vi "Play Path.vi"(7 "Description":string, 8 "Command Info In":T5, 11 "Path stuff":T4 {"Limits"."Limits"."StoopidFast (fps)" min=0.0; "Limits"."Limits"."Jerk (fps^3)" min=0.0 step=1.0; "Limits"."Limits"."Accel (fps^2)" min=0.0; "Limits"."Limits"."Velocity (fps)" min=0.0}) -> (0 "Command Info Out":T5)   [LabVIEW 2019]
doc: "This VI notifies the subsystem to the new setpoint."
uses:
  <vilib>/Rock Robotics/WPI/Framework/Command Status Info.ctl
  <vilib>/Rock Robotics/WPI/Framework/Completion Status.ctl
  <vilib>/Rock Robotics/WPI/Framework/Completion Notifier.ctl
  Support Code/Single Cmd Info.ctl
  <vilib>/picture/picture.llb/imagedata.ctl
  Support Code/types/Limits.ctl
  Implementation/Drive Operations.ctl
  Implementation/Drive Setpoints.ctl
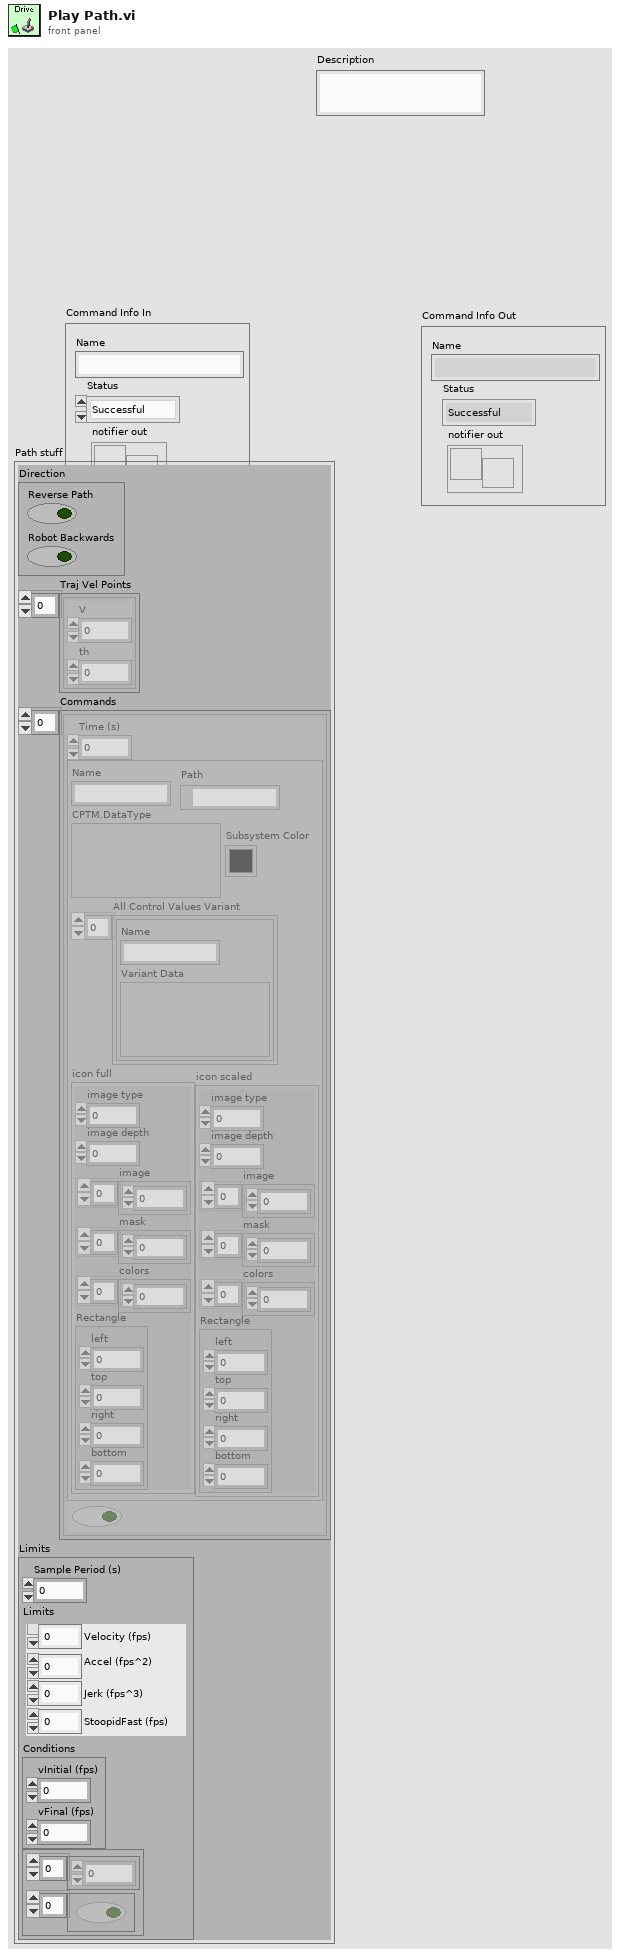
[diagram p1: front panel]
types:
  T1 = typedef "Single Cmd Info.ctl" = cluster{"Name":string, "CPTM.DataType":variant, "All Control Values Variant":cluster{"Name":string, "Variant Data":variant}[], "icon full":T2, "icon scaled":T2, "Path":path, "Subsystem Color":u32}
  T2 = typedef "imagedata.ctl" = cluster{"image type":i32, "image depth":i32, "image":u8[], "mask":u8[], "colors":u32[], "Rectangle":cluster{"left":i16, "top":i16, "right":i16, "bottom":i16}}
  T3 = typedef "Limits.ctl" = cluster{"Velocity (fps)":dbl, "Accel (fps^2)":dbl, "Jerk (fps^3)":dbl, "StoopidFast (fps)":dbl}
  T4 = cluster{"Direction":cluster{"Reverse Path":bool, "Robot Backwards":bool}, "Traj Vel Points":cluster{"V":dbl, "th":dbl}[], "Commands":cluster{"Time (s)":dbl, T1, bool}[], "Limits":cluster{"Sample Period (s)":dbl, "Limits":T3, "Conditions":cluster{"vInitial (fps)":dbl, "vFinal (fps)":dbl}, cluster{dbl[], bool[]}}}
  T5 = typedef "Command Status Info.ctl" = cluster{"Name":string, "Status":T6, "notifier out":T7}
  T6 = typedef "Completion Status.ctl" = enum16{"Successful", "Aborted", "Incomplete"}
  T7 = typedef "Completion Notifier.ctl" = refnum<notifier>
  T8 = typedef "Drive Operations.ctl" = enum16{"Reserve", "Read Current", "Immediate", "Play Path"}
  T9 = typedef "Drive Setpoints.ctl" = cluster{"Operation":T8, "Setpoints":cluster{"Left Setpoint":dbl, "Right Setpoint":dbl}, "Path stuff":cluster{"Direction":cluster{"Reverse Path":bool, "Robot Backwards":bool}, "Traj Vel Points":cluster{"V":dbl, "th":dbl}[], "Commands":cluster{"Time (s)":dbl, T1, bool}[], "Limits":cluster{"Sample Period (s)":dbl, "Limits":T3, "Conditions":cluster{"vInitial (fps)":dbl, "vFinal (fps)":dbl}, cluster{dbl[], bool[]}}}}
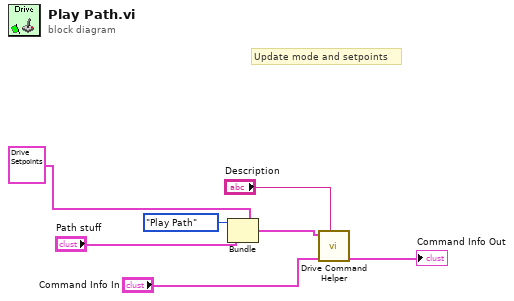
[diagram p0: block diagram]
diagram:
  # "Update mode and setpoints"
  n1 = Bundle(cluster=T9 {"Operation"=enum."Reserve", "Setpoints"={"Left Setpoint"=0.0, "Right Setpoint"=0.0}, "Path stuff"={"Direction"={"Reverse Path"=FALSE, "Robot Backwards"=FALSE}, "Traj Vel Points"=[], "Commands"=[], "Limits"={"Sample Period (s)"=0.0, "Limits"={"Velocity (fps)"=0.0, "Accel (fps^2)"=0.0, "Jerk (fps^3)"=0.0, "StoopidFast (fps)"=0.0}, "Conditions"={"vInitial (fps)"=0.0, "vFinal (fps)"=0.0}, {[], []}}}} ("output cluster"), "Operation"=Drive_Operations."Play Path", "Path stuff"="Path stuff") -> (w1:T9)  [unwired: 1 in]
  n2 = call "Drive Command Helper.vi"("Description"="Description", "Command Info In"="Command Info In", "SubSystem Data"=w1) -> ("Command Info Out"=→"Command Info Out":T5)  [unwired: 6 in, 2 out]
